vi "ArmCurlSystem.vi"(8 "Reset Encoder":bool, 9 "Arm Down":bool, 10 "Arm Up":bool, 11 "Shoulder Speed":dbl) -> ()   [LabVIEW 2018]
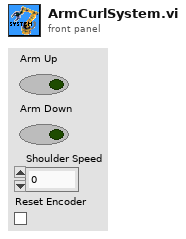
[diagram p1: front panel]
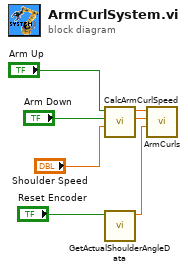
[diagram p0: block diagram]
diagram:
  n1 = call "CalcArmCurlSpeed.vi"("Curl Speed"="Shoulder Speed", "Arm Down"="Arm Down", "Arm Up"="Arm Up") -> ("Arm Speed"=w7:dbl, "Shoulder Speed"=w2:dbl)  [unwired: 7 in]
  n2 = call "GetActualShoulderAngleData.vi"("Reset Encoder"="Reset Encoder") -> ("Encoder Angle (deg)"=w1:dbl)  [unwired: 9 in, 1 out]
  n3 = call "ArmCurls.vi"("Actual Shoulder Angle (deg)"=w1, "Arm Speed"=w7, "shoulder speed (deg/s)"=w2) -> ()  [unwired: 9 in]
